vi "HovaCAL auf Fehler Testen.vi"(8 "error in (no error)":errorcluster caption="Fehler (Eingang, kein Fehler)") -> (0 "error out":errorcluster caption="Fehler (Ausgang)", 2 "Error":bool, 3 "LNI Error Ausgangs-Cluster":T1)   [LabVIEW 2020, in "Linearisierung v2.lvlib" / "Gasteiler.lvlib" / "HovaCAL_Interface.lvlib"]
uses:
  HovaCAL_Interface.lvlib
  LIN ErrorCluster.ctl
  Aktion FGV Stoerungen sammeln und auswerten.ctl
  Kommunikation/Aktion_FGV_HovaCAL_Interface_GetData.ctl
  Kommunikation/Aktion_FGV_HovaCAL_Interface_SetData.ctl
  Kommunikation/Kommunikation.lvlib
  Linearisierung v2.lvlib
  SpanEinstellungen/SpanEinstellungen.lvlib
  Helper/Helper.lvlib
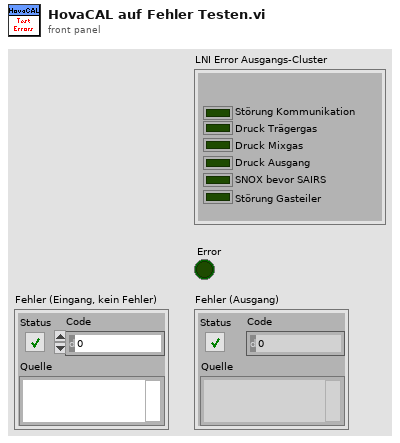
[diagram p1: front panel]
types:
  T1 = typedef "Linearisierung v2.lvlib/LIN ErrorCluster.ctl" = cluster{"Störung Kommunikation":bool, "Pressure carrier gas":bool, "Pressure diluted gas":bool, "Outlet Pressure":bool, "SNOX before SAIR":bool, "Störung Gasteiler":bool}
  T2 = typedef "Linearisierung v2.lvlib/Gasteiler.lvlib/HovaCAL_Interface.lvlib/Kommunikation.lvlib/Aktion_FGV_HovaCAL_Interface_GetData.ctl" = enum16{"lesen", "SystemInfo", "MFC Info", "actual Values", "Limits", "first contact", "reset after read"}
  T3 = typedef "Linearisierung v2.lvlib/Aktion FGV Stoerungen sammeln und auswerten.ctl" = enum16{"init", "lesen", "error", "prüfen", "reset error", "abbrechen", "fortsetzen", "neustart", "Bedientasten reset"}
  T4 = typedef "Linearisierung v2.lvlib/Gasteiler.lvlib/HovaCAL_Interface.lvlib/Controls.lvlib/Info Cluster.ctl" = cluster{"device":string, "version":string, "number of mfc":i32, "number of pumps":i32, "number of temp controllers":i32, "number of mfs":i32, "number of balances":i32}
  T5 = cluster{"reagent conc":dbl, "reagent conc dry":dbl, "water conc":dbl, "water conc dry":dbl, "speed":dbl}[]
  T6 = typedef "Linearisierung v2.lvlib/Gasteiler.lvlib/HovaCAL_Interface.lvlib/Controls.lvlib/MFC Output plus Input Output Concentrations.ctl" = cluster{"Input Concentration":dbl, "Output Setpoint":dbl, "output concentration":dbl, "output concentration dry":dbl, "flow actual":dbl, "flow expected":dbl}
  T7 = typedef "Linearisierung v2.lvlib/Gasteiler.lvlib/HovaCAL_Interface.lvlib/Kommunikation.lvlib/Aktion_FGV_HovaCAL_Interface_SetData.ctl" = enum16{"lesen", "Konzentrationen", "Pumpen Parameter", "Pumpe Konzentration", "Pumpe run", "Temperaturen", "Fluss", "Limits", "init"}
  T8 = cluster{"input concentration setpoint":dbl, "output concentration setpoint":dbl}[]
  T9 = cluster{"input concentration setpoint":dbl, "output concentration setpoint":dbl}
  T10 = typedef "Linearisierung v2.lvlib/Gasteiler.lvlib/HovaCAL_Interface.lvlib/Controls.lvlib/Pump Concentration Mode.ctl" = i32
  T11 = typedef "Linearisierung v2.lvlib/Gasteiler.lvlib/HovaCAL_Interface.lvlib/Controls.lvlib/Reagent.ctl" = i32
  T12 = cluster{"concentratio mode":T10, "Reagent":T11, "Molarity":dbl, "density":dbl, "syringe":dbl, "pump_a":dbl}[]
  T13 = typedef "Linearisierung v2.lvlib/Gasteiler.lvlib/HovaCAL_Interface.lvlib/Controls.lvlib/Pump Concentration.ctl" = cluster{"reagent conc SP":dbl, "water conc SP":dbl}
  T14 = typedef "Linearisierung v2.lvlib/Gasteiler.lvlib/HovaCAL_Interface.lvlib/Controls.lvlib/Pump Dry Mode.ctl" = i32
  T15 = typedef "Linearisierung v2.lvlib/Gasteiler.lvlib/HovaCAL_Interface.lvlib/Controls.lvlib/Pump Control Mode.ctl" = u32
  T16 = cluster{"running?":bool, "dry mode":T14, "control mode":T15}
  T17 = cluster{"reagent conc":dbl, "reagent conc dry":dbl, "water conc":dbl, "water conc dry":dbl, "speed":dbl}
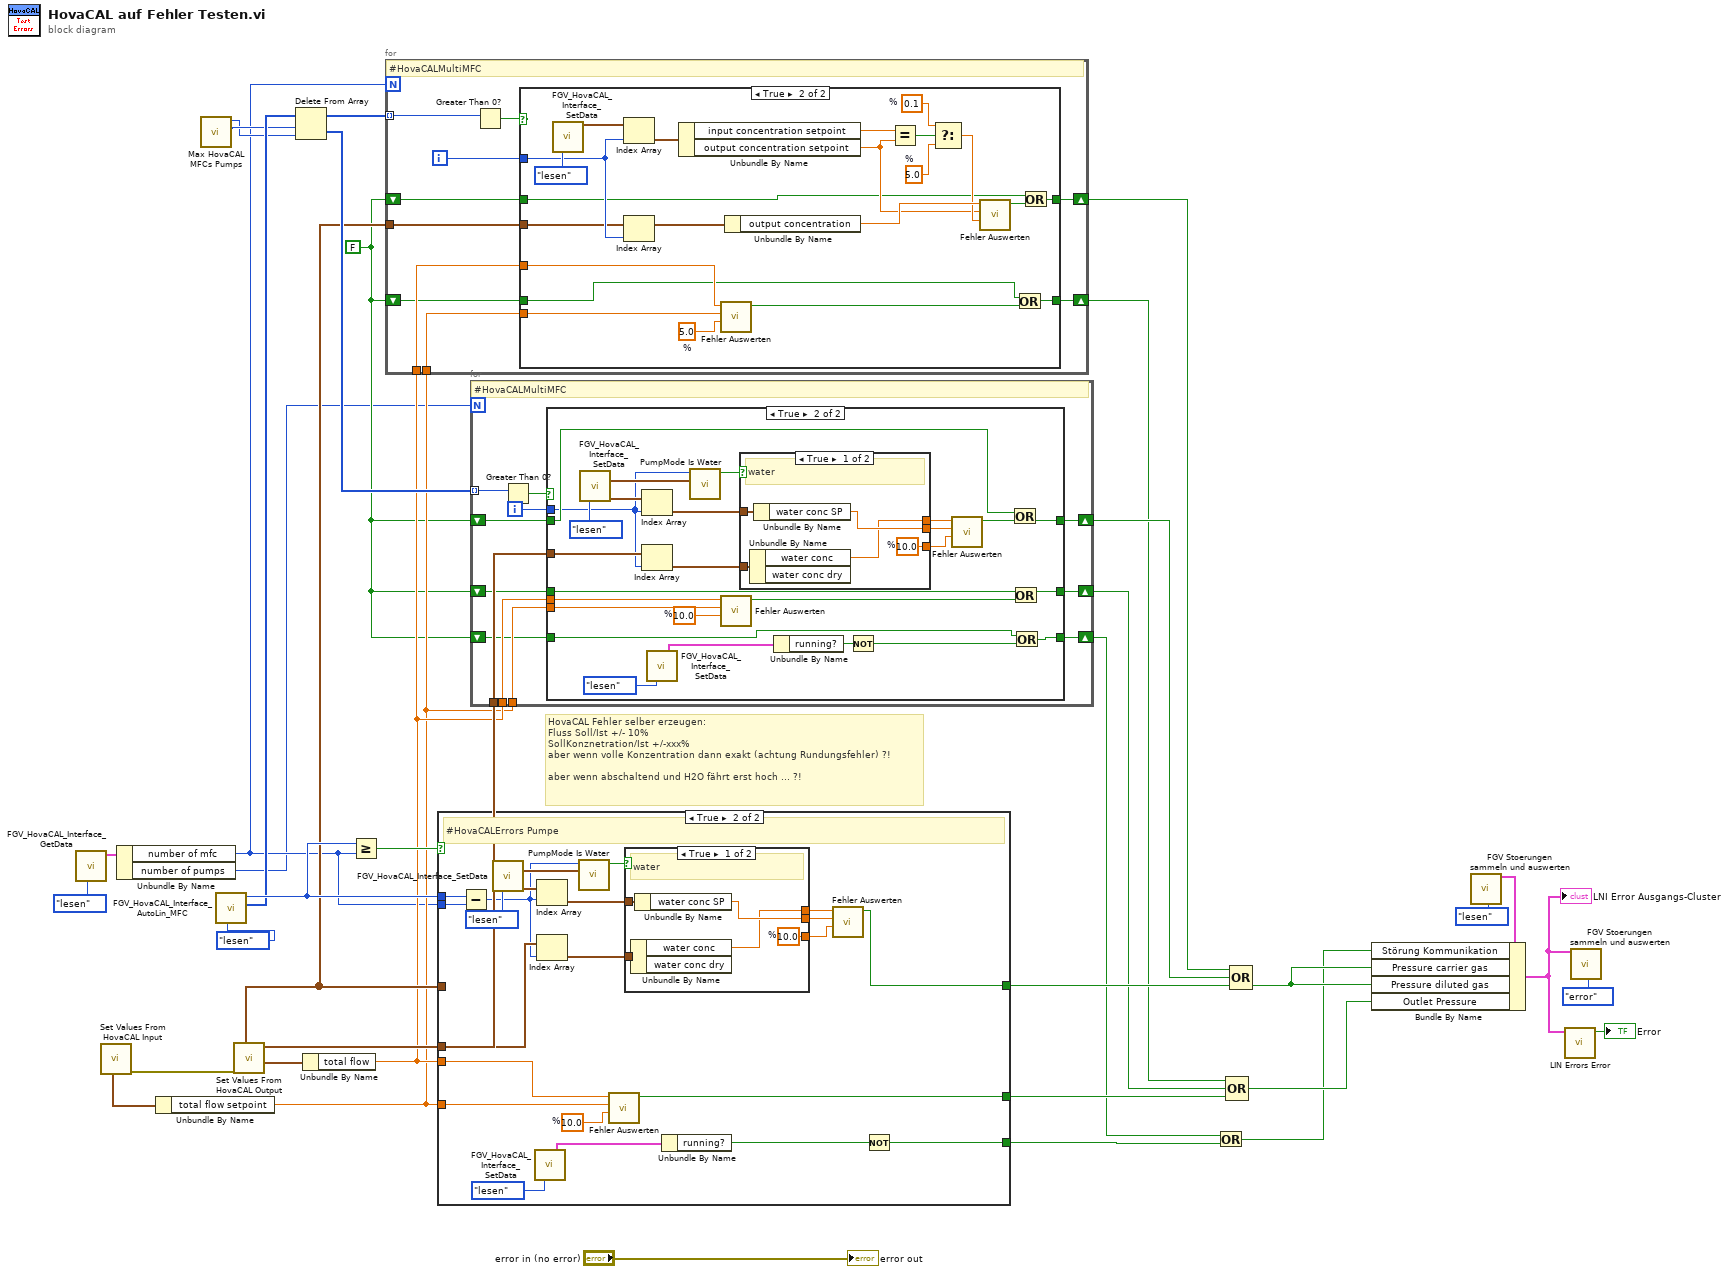
[diagram p0: block diagram]
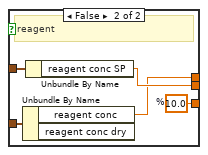
[diagram p3: hidden frame]
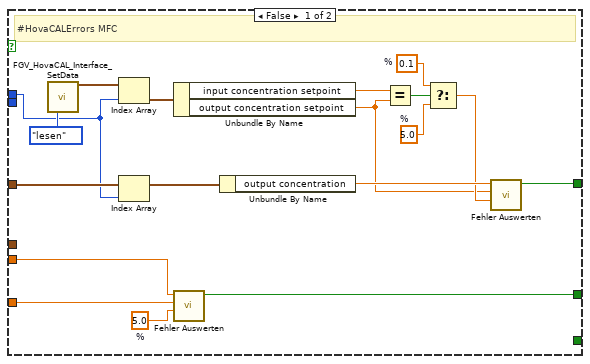
[diagram p5: hidden frame]
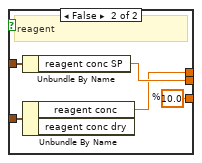
[diagram p6: hidden frame]
diagram:
  w13 = FALSE ("Error")
  # "HovaCAL Fehler selber erzeugen:\nFluss Soll/Ist +/- 10% \nSollKonznetration/Ist +/-xxx% \naber wenn volle Konzentration dann exakt (achtung Rundungsfehler) ?!\n\naber wenn abschaltend und H2O fährt erst hoch ... ?!"
  n1 = call "FGV_HovaCAL_Interface_GetData.vi"("Aktion"=Aktion_FGV_HovaCAL_Interface_GetData."lesen") -> ("System Cluster out"=w28:T4)  [unwired: 6 in, 4 out]
  n2 = call "Set Values From HovaCAL Input.vi"() -> ("error out"=w33:errorcluster, "Flow Input Cluster"=w32:cluster{"total flow setpoint":dbl})  [unwired: 3 in, 7 out]
  n3 = Unbundle By Name(w28) -> ("number of mfc"=w2:i32, "number of pumps"=w1:i32)
  n4 = Unbundle By Name(w32) -> ("total flow setpoint"=w14:dbl)
  n5 = call "Max HovaCAL MFCs Pumps.vi"() -> ("max Pumps"=w4:i32, "max MFCs"=w3:i32)  [unwired: 10 in]
  n6 = call "FGV_HovaCAL_Interface_AutoLin_MFC.vi"("Aktion"=enum16{"lesen", "schreiben"}."lesen") -> ("MFV Komponente fix out"=w20:u16[], "AutoLin MFC out"=w21:u16)  [unwired: 7 in, 2 out]
  n7 = call "Set Values From HovaCAL Output.vi"("error in (no error)"=w33) -> ("Cluster.Flow Output Cluster (Ausgang)"=w31:cluster{"total flow":dbl}, "Cluster.Pump Concentrations-Cluster"=w17:T5, "MFC Input/Output Concentrations (Ausgang)"=w16:T6[])  [unwired: 8 out]
  n8 = Delete From Array(array=w20, length=w4, index=w3) -> (deleted portion=w18:u16[], array with subset deleted=w19:u16[])
  n9 = Unbundle By Name(w31) -> ("total flow"=w15:dbl)
  n10 = Greater Or Equal?(x=w21, y=w2) -> (x >= y?=w27:bool)
  n11 = for {
    N: w2 -> [_]
    tunnel: w19 -> [w47] mode=indexing
    tunnel: w16 -> [w44]
    tunnel: w15 -> [w43]
    tunnel: w14 -> [w42]
    shift-right: [w41] -> w10
    shift-left: w13 -> [w39]
    shift-right: [w40] -> w7
    shift-left: w13 -> [w38]
    i -> [w45]
    # "#HovaCALMultiMFC"
    n12 = Greater Than 0?(x=w47) -> (x > 0?=w46:bool)
    n13 = case shown="True" w46 {
      tunnel: w45 -> [_ w59]
      tunnel: w44 -> [_ w58]
      tunnel: w43 -> [_ w57]
      tunnel: w42 -> [_ w56]
      tunnel: [w49 w53] -> w41
      tunnel: [w48 w51] -> w40
      tunnel: w39 -> [w49 w52]
      tunnel: w38 -> [w48 w50]
      frame False {
      }
      frame True {
        w60 = 5.0  # %
        w64 = 0.1  # %
        w63 = 5.0  # %
        n14 = call "FGV_HovaCAL_Interface_SetData.vi"("Aktion"=Aktion_FGV_HovaCAL_Interface_SetData."lesen") -> ("Set Values Cluster out"=w70:T8)  [unwired: 8 in, 6 out]
        n15 = Index Array(array=w70, index=w59) -> (element=w69:T9)
        n16 = Index Array(array=w58, index=w59) -> (element=w68:T6)
        n17 = Unbundle By Name(w69) -> ("input concentration setpoint"=w66:dbl, "output concentration setpoint"=w61:dbl)
        n18 = call "Fehler Auswerten.vi"("Max Fehler in %"=w60, "setpoint"=w56, "output"=w57) -> ("Error"=w54:bool)  [unwired: 8 in]
        n19 = Unbundle By Name(w68) -> ("output concentration"=w67:dbl)
        n20 = Equal?(x=w66, y=w61) -> (x = y?=w65:bool)
        n21 = Select(t=w64, s=w65, f=w63) -> (s? t:f=w62:dbl)
        n22 = call "Fehler Auswerten.vi"("Max Fehler in %"=w62, "setpoint"=w61, "output"=w67) -> ("Error"=w55:bool)  [unwired: 8 in]
        n23 = Or(x=w50, y=w54) -> (x .or. y?=w51:bool)
        n24 = Or(x=w52, y=w55) -> (x .or. y?=w53:bool)
      }
    }
  }
  n25 = case shown="True" w27 {
    tunnel: w15 -> [w84 w101]
    tunnel: w14 -> [w83 w100]
    tunnel: w16 -> [w86 _]
    tunnel: w17 -> [_ w106]
    tunnel: [_ w103] -> w26
    tunnel: [w81 w99] -> w25
    tunnel: [w79 w95] -> w24
    tunnel: w2 -> [_ w94]
    tunnel: w21 -> [w72 w93]
    frame False {
      w76 = 0.1  # %
      w75 = 5.0  # %
      w82 = 5.0  # %
      # "#HovaCALErrors MFC"
      n26 = call "FGV_HovaCAL_Interface_SetData.vi"("Aktion"=Aktion_FGV_HovaCAL_Interface_SetData."lesen") -> ("Set Values Cluster out"=w88:T8)  [unwired: 8 in, 6 out]
      n27 = Index Array(array=w88, index=w72) -> (element=w87:T9)
      n28 = Index Array(array=w86, index=w72) -> (element=w85:T6)
      n29 = Unbundle By Name(w87) -> ("input concentration setpoint"=w78:dbl, "output concentration setpoint"=w73:dbl)
      n30 = call "Fehler Auswerten.vi"("Max Fehler in %"=w82, "setpoint"=w83, "output"=w84) -> ("Error"=w81:bool)  [unwired: 8 in]
      n31 = Unbundle By Name(w85) -> ("output concentration"=w80:dbl)
      n32 = Equal?(x=w78, y=w73) -> (x = y?=w77:bool)
      n33 = Select(t=w76, s=w77, f=w75) -> (s? t:f=w74:dbl)
      n34 = call "Fehler Auswerten.vi"("Max Fehler in %"=w74, "setpoint"=w73, "output"=w80) -> ("Error"=w79:bool)  [unwired: 8 in]
    }
    frame True {
      w102 = 10.0  # %
      # "#HovaCALErrors Pumpe"
      n35 = Subtract(x=w93, y=w94) -> (x-y=w91:i32)
      n36 = call "FGV_HovaCAL_Interface_SetData.vi"("Aktion"=Aktion_FGV_HovaCAL_Interface_SetData."lesen") -> ("PumpMode-Cluster out"=w92:T12, "Pump Concentrations-Cluster out"=w110:T13[])  [unwired: 8 in, 5 out]
      n37 = call "FGV_HovaCAL_Interface_SetData.vi"("Aktion"=Aktion_FGV_HovaCAL_Interface_SetData."lesen") -> ("PumpModeGeneral-Cluster out"=w108:T16)  [unwired: 8 in, 6 out]
      n38 = Index Array(array=w110, index=w91) -> (element=w109:T13)
      n39 = Index Array(array=w106, index=w91) -> (element=w105:T17)
      n40 = call "PumpMode Is Water.vi"("PumpMode-Cluster out"=w92, "Numerisch"=w91) -> ("is Water"=w90:bool)  [unwired: 9 in]
      n41 = call "Fehler Auswerten.vi"("Max Fehler in %"=w102, "setpoint"=w100, "output"=w101) -> ("Error"=w99:bool)  [unwired: 8 in]
      n42 = case shown="True" w90 {
        tunnel: w109 -> [w116 w121]
        tunnel: w105 -> [w115 w120]
        tunnel: [w114 w119] -> w98
        tunnel: [w113 w118] -> w97
        tunnel: [w112 w117] -> w96
        frame True {
          w114 = 10.0  # %
          # "water"
          n43 = Unbundle By Name(w115) -> ("water conc"=w112:dbl)  [unwired: 1 out]
          n44 = Unbundle By Name(w116) -> ("water conc SP"=w113:dbl)
        }
        frame False {
          w119 = 10.0  # %
          # "reagent"
          n45 = Unbundle By Name(w121) -> ("reagent conc SP"=w118:dbl)
          n46 = Unbundle By Name(w120) -> ("reagent conc"=w117:dbl)  [unwired: 1 out]
        }
      }
      n47 = Unbundle By Name(w108) -> ("running?"=w104:bool)
      n48 = call "Fehler Auswerten.vi"("Max Fehler in %"=w98, "setpoint"=w97, "output"=w96) -> ("Error"=w95:bool)  [unwired: 8 in]
      n49 = Not(x=w104) -> (.not. x?=w103:bool)
    }
  }
  n50 = for {
    N: w1 -> [_]
    tunnel: w18 -> [w133] mode=indexing
    tunnel: w17 -> [w130]
    shift-right: [w129] -> w11
    shift-left: w13 -> [w124]
    tunnel: w15 -> [w126]
    tunnel: w14 -> [w125]
    shift-right: [w128] -> w8
    shift-left: w13 -> [w123]
    shift-right: [w127] -> w5
    shift-left: w13 -> [w122]
    i -> [w131]
    # "#HovaCALMultiMFC"
    n51 = Greater Than 0?(x=w133) -> (x > 0?=w132:bool)
    n52 = case shown="True" w132 {
      tunnel: w131 -> [_ w138]
      tunnel: w130 -> [_ w156]
      tunnel: [w136 w147] -> w129
      tunnel: w126 -> [_ w150]
      tunnel: w125 -> [_ w149]
      tunnel: [w135 w144] -> w128
      tunnel: [w134 w141] -> w127
      tunnel: w124 -> [w136 w145]
      tunnel: w123 -> [w135 w142]
      tunnel: w122 -> [w134 w140]
      frame False {
      }
      frame True {
        w151 = 10.0  # %
        n53 = call "FGV_HovaCAL_Interface_SetData.vi"("Aktion"=Aktion_FGV_HovaCAL_Interface_SetData."lesen") -> ("PumpMode-Cluster out"=w139:T12, "Pump Concentrations-Cluster out"=w162:T13[])  [unwired: 8 in, 5 out]
        n54 = Index Array(array=w162, index=w138) -> (element=w161:T13)
        n55 = Index Array(array=w156, index=w138) -> (element=w160:T17)
        n56 = call "FGV_HovaCAL_Interface_SetData.vi"("Aktion"=Aktion_FGV_HovaCAL_Interface_SetData."lesen") -> ("PumpModeGeneral-Cluster out"=w154:T16)  [unwired: 8 in, 6 out]
        n57 = call "PumpMode Is Water.vi"("PumpMode-Cluster out"=w139, "Numerisch"=w138) -> ("is Water"=w137:bool)  [unwired: 9 in]
        n58 = call "Fehler Auswerten.vi"("Max Fehler in %"=w151, "setpoint"=w149, "output"=w150) -> ("Error"=w143:bool)  [unwired: 8 in]
        n59 = case shown="True" w137 {
          tunnel: w161 -> [w167 w172]
          tunnel: w160 -> [w166 w171]
          tunnel: [w165 w170] -> w159
          tunnel: [w164 w169] -> w158
          tunnel: [w163 w168] -> w157
          frame True {
            w165 = 10.0  # %
            # "water"
            n60 = Unbundle By Name(w166) -> ("water conc"=w163:dbl)  [unwired: 1 out]
            n61 = Unbundle By Name(w167) -> ("water conc SP"=w164:dbl)
          }
          frame False {
            w170 = 10.0  # %
            # "reagent"
            n62 = Unbundle By Name(w171) -> ("reagent conc"=w168:dbl)  [unwired: 1 out]
            n63 = Unbundle By Name(w172) -> ("reagent conc SP"=w169:dbl)
          }
        }
        n64 = Unbundle By Name(w154) -> ("running?"=w152:bool)
        n65 = Not(x=w152) -> (.not. x?=w148:bool)
        n66 = call "Fehler Auswerten.vi"("Max Fehler in %"=w159, "setpoint"=w158, "output"=w157) -> ("Error"=w155:bool)  [unwired: 8 in]
        n67 = Or(x=w145, y=w155) -> (x .or. y?=w147:bool)
        n68 = Or(x=w142, y=w143) -> (x .or. y?=w144:bool)
        n69 = Or(x=w140, y=w148) -> (x .or. y?=w141:bool)
      }
    }
  }
  n70 = Or(x=w5, y=w26) -> (x .or. y?=w6:bool)
  n71 = Compound Arithmetic op=OR ("Mehrfacharithmetik")(w7, w8, w25) -> (w9:bool)
  n72 = Compound Arithmetic op=OR ("Mehrfacharithmetik")(w10, w11, w24) -> (w12:bool)
  n73 = call "FGV Stoerungen sammeln und auswerten.vi"("Aktion"=Aktion_FGV_Stoerungen_sammeln_und_auswerten."lesen") -> ("Errors"=w34:T1)  [unwired: 12 in, 6 out]
  n74 = Bundle By Name(cluster=w34, "Störung Kommunikation"=w6, "Pressure carrier gas"=w12, "Pressure diluted gas"=w12, "Outlet Pressure"=w9) -> (w23:T1)
  "LNI Error Ausgangs-Cluster" <- w23
  n75 = call "LIN Errors Error.vi"("Errors"=w23) -> ("Error"=→"Error":bool)  [unwired: 10 in]
  n76 = call "FGV Stoerungen sammeln und auswerten.vi"("Errors"=w23, "Aktion"=Aktion_FGV_Stoerungen_sammeln_und_auswerten."error") -> ()  [unwired: 11 in, 7 out]
  "error out" <- "error in (no error)"
